vi "Prompt for Step--Init UI.vi"(8 "error in (no error)":errorcluster, 10 "Control Ref Map":map{string, refnum<vi>}(c390), 11 "Numeric Assertion in":refnum<class "Numeric Assertion.lvclass">) -> (0 "error out":errorcluster, 3 "Numeric Assertion out":refnum<class "Numeric Assertion.lvclass">)   [LabVIEW 2020, in "MacroAssert.lvlib" / "Numeric Assertion.lvclass"]
doc: "Initializes the user interface within the \"Prompt for Step\" VI."
uses:
  Numeric Assertion.lvclass
  5ba077b8-b607-459d-98e5-8a29527f14dd.vi
  b760b8db-bf85-4f92-9ee9-d68b04e20580.vi
  Support/Get Control Reference by Label (1D STR).vi
  <vilib>/Utility/error.llb/Error Cluster From Error Code.vi
  Assertion Step/Assertion Step.lvclass
  MacroAssert.lvlib
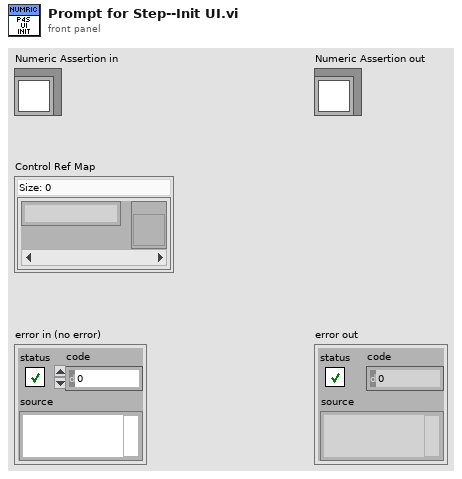
[diagram p1: front panel]
types:
  T1 = typedef "MacroAssert.lvlib/Numeric Assertion.lvclass/Numeric Assertion Type.ctl" = enum16{"Numeric Ctl Value", "Ctl Width Property", "Ctl Height Property", "VI Width", "VI Height", "Window Width", "Window Height"}
  T2 = typedef "MacroAssert.lvlib/Numeric Assertion.lvclass/Numeric Comparator.ctl" = enum16{"Equals", "Is greater than", "Is greater than or equal to", "Is less than", "Is less than or equal to", "Does not equal"}
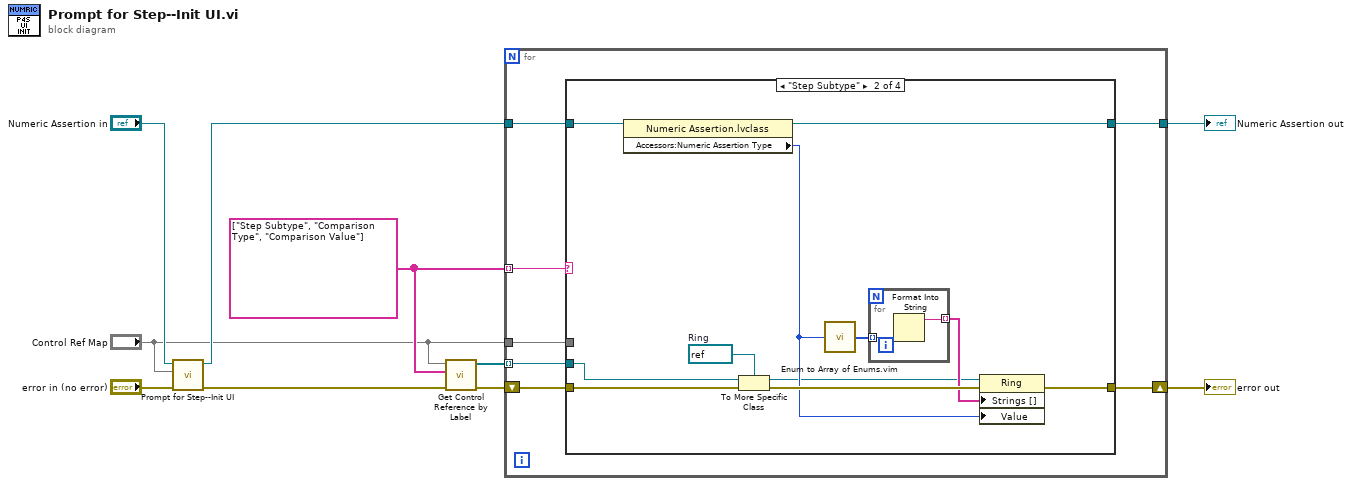
[diagram p0: block diagram]
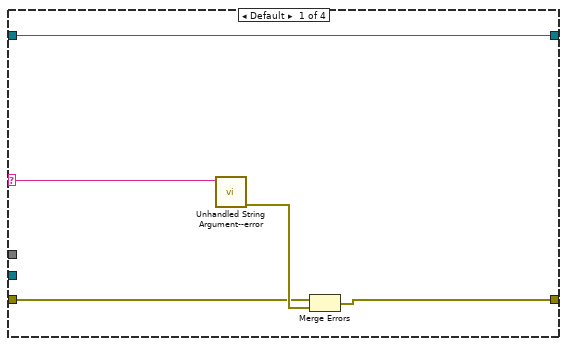
[diagram p2: hidden frame]
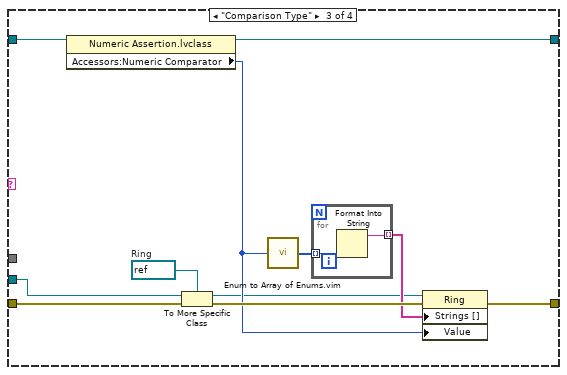
[diagram p3: hidden frame]
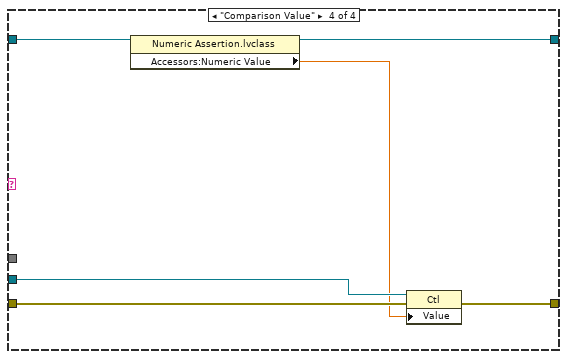
[diagram p4: hidden frame]
diagram:
  w9 = string[] ["Step Subtype", "Comparison Type", "Comparison Value"]
  n1 = call-parent "Prompt for Step--Init UI.vi"("error in (no error)"="error in (no error)", "Control Ref Map"="Control Ref Map", "Assertion Step in"="Numeric Assertion in") -> ("error out"=w4:errorcluster, "Assertion Step out"=w2:refnum<class "Numeric Assertion.lvclass">)  [unwired: 7 in]
  n2 = call-poly "Get Control Reference by Label.vi"("error in (no error)"=w4, "Control Names"=w9, "Control Ref Map"="Control Ref Map") -> ("error out"=w10:errorcluster, "Control Refs"=w8:refnum<vi>[])  [unwired: 6 in, 1 out]
  n3 = for {
    tunnel: w2 -> [w15]
    tunnel: [w13] -> w6
    tunnel: w9 -> [w16] mode=indexing
    tunnel: w8 -> [w14] mode=indexing
    shift-right: [w12] -> w7
    shift-left: w10 -> [w17]
    tunnel: "Control Ref Map" -> [w11]
    n4 = case shown="\"Step Subtype\"" w16 {
      selector: w16 -> [w19 _ _ _]
      tunnel: w17 -> [w20 w27 w40 w51]
      tunnel: w15 -> [w22 w28 w41 w54]
      tunnel: w14 -> [_ w26 w39 w52]
      tunnel: [w22 w23 w36 w53] -> w13
      tunnel: [w18 w25 w38 w49] -> w12
      tunnel: w11 -> [_ _ _ _]
      frame Default {
        n5 = call "Unhandled String Argument--error.vi"("Argument"=w19) -> ("error out"=w21:errorcluster)  [unwired: 10 in]
        n6 = Merge Errors(w20, w21) -> (w18:errorcluster)
      }
      frame "Step Subtype" {
        w31 = refnum<vi> refnum  # Ring
        n7 = property class="Numeric Assertion.lvclass"(reference=w28) -> (reference out=w23:refnum<class "Numeric Assertion.lvclass">, "Accessors:Numeric Assertion Type"=w30:T1)  [unwired: 1 in, 1 out]
        n8 = To More Specific Class(target class=w31, reference=w26, error in=w27) -> (specific class reference=w24:refnum<vi>, error out=w32:errorcluster)
        n9 = call "Enum to Array of Enums.vim"("enum"=w30) -> ("array of enums"=w33:T1[])
        n10 = for {
          tunnel: w33 -> [w35] mode=indexing
          tunnel: [w34] -> w29 mode=indexing
          n11 = Format Into String(w35) -> (resulting string=w34:string)  [unwired: 3 in, 1 out]
        }
        n12 = property class="Ring"(reference=w24, error in=w32, "Strings []"=w29, "Value"=w30) -> (error out=w25:errorcluster)  [unwired: 1 out]
      }
      frame "Comparison Type" {
        w44 = refnum<vi> refnum  # Ring
        n13 = property class="Numeric Assertion.lvclass"(reference=w41) -> (reference out=w36:refnum<class "Numeric Assertion.lvclass">, "Accessors:Numeric Comparator"=w43:T2)  [unwired: 1 in, 1 out]
        n14 = To More Specific Class(target class=w44, reference=w39, error in=w40) -> (specific class reference=w37:refnum<vi>, error out=w45:errorcluster)
        n15 = call "Enum to Array of Enums.vim"("enum"=w43) -> ("array of enums"=w46:T2[])
        n16 = for {
          tunnel: w46 -> [w48] mode=indexing
          tunnel: [w47] -> w42 mode=indexing
          n17 = Format Into String(w48) -> (resulting string=w47:string)  [unwired: 3 in, 1 out]
        }
        n18 = property class="Ring"(reference=w37, error in=w45, "Strings []"=w42, "Value"=w43) -> (error out=w38:errorcluster)  [unwired: 1 out]
      }
      frame "Comparison Value" {
        n19 = property class="Numeric Assertion.lvclass"(reference=w54) -> (reference out=w53:refnum<class "Numeric Assertion.lvclass">, "Accessors:Numeric Value"=w50:dbl)  [unwired: 1 in, 1 out]
        n20 = property class="Ctl"(reference=w52, error in=w51, "Value"=w50) -> (error out=w49:errorcluster)  [unwired: 1 out]
      }
    }
  }
  "error out" <- w7
  "Numeric Assertion out" <- w6
